vi "DetectPeaks.vi"(10 "Y":dbl[](array[numeric]), 11 "X":dbl[](array[numeric])) -> (2 "Amplitudes":dbl[](array[numeric]), 3 "Locations":dbl[](array[numeric]))   [LabVIEW 2013]
uses:
  Global.vi
  <vilib>/Analysis/NI_AAL_SigProc.lvlib
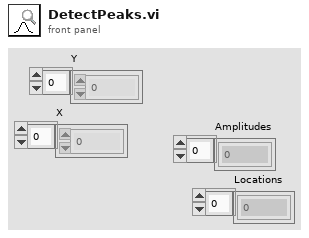
[diagram p1: front panel]
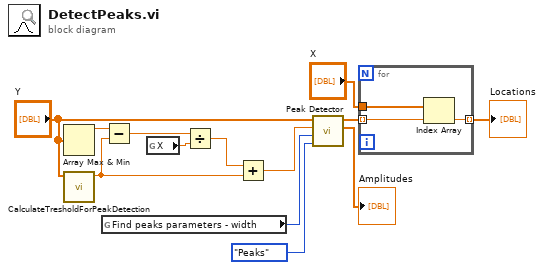
[diagram p0: block diagram]
diagram:
  n1 = Array Max & Min(array="Y") -> (max value=w6:dbl)  [unwired: 3 out]
  n2 = call "CalculateTresholdForPeakDetection.vi"("Array"="Y") -> ("Average"=w3:dbl)  [unwired: 10 in]
  n3 = global read "Global.vi" "Find peaks parameters - width"() -> (w8:i32)
  n4 = Subtract(x=w6, y=w3) -> (x-y=w4:dbl)
  n5 = global read "Global.vi" "X"() -> (w5:dbl)
  n6 = Divide(x=w4, y=w5) -> (x/y=w2:dbl)
  n7 = Add(x=w2, y=w3) -> (x+y=w1:dbl)
  n8 = call <vilib>:"Peak Detector.vi"("peaks/valleys"=enum32{"Peaks", "Valleys"}."Peaks", "width"=w8, "threshold"=w1, "X"="Y") -> ("Amplitudes"=→"Amplitudes":dbl[], "Locations"=w11:dbl[])  [unwired: 3 in, 3 out]
  n9 = for {
    tunnel: w11 -> [w15] mode=indexing
    tunnel: "X" -> [w16]
    tunnel: [w14] -> w9 mode=indexing
    n10 = Index Array(array=w16, index=w15) -> (element=w14:dbl)
  }
  "Locations" <- w9
